vi "FPGA Read.vi"(8 "error in (no error)":errorcluster, 11 "FPGA VI Reference IN":refnum<k20>) -> (0 "error out":errorcluster, 1 "DIO OUT":bool[](array[boolean]), 2 "Raw Ball Voltages OUT":sgl[](array[numeric]), 3 "FPGA VI Reference OUT":refnum<k20>)   [LabVIEW 2018]
uses:
  <vilib>/Utility/error.llb/Error Cluster From Error Code.vi
  <vilib>/rvi/errors/niLvFpgaAdjustHostInterfaceError.vi
  <vilib>/rvi/interface/nirviReadWriteControl/nirviReadWriteControl.xnode
  NiFpgaLv.dll
  <vilib>/rvi/interface/Simulation/niFpgaSimulationCallBeginRW.vi
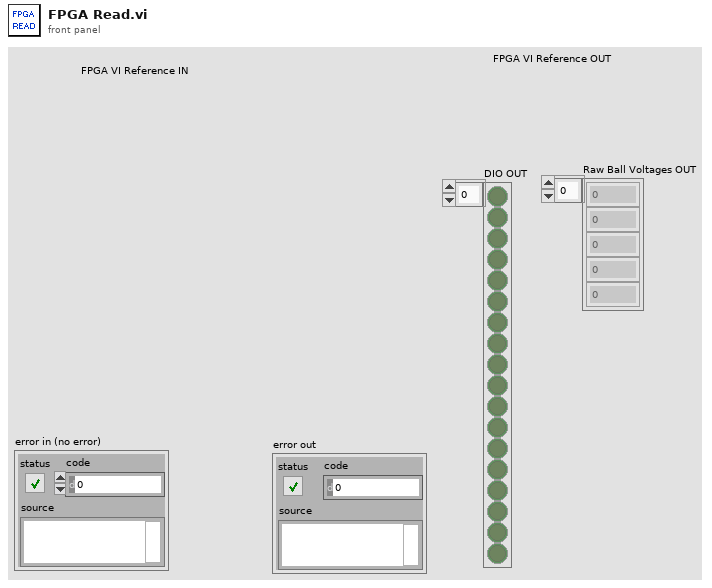
[diagram p1: front panel]
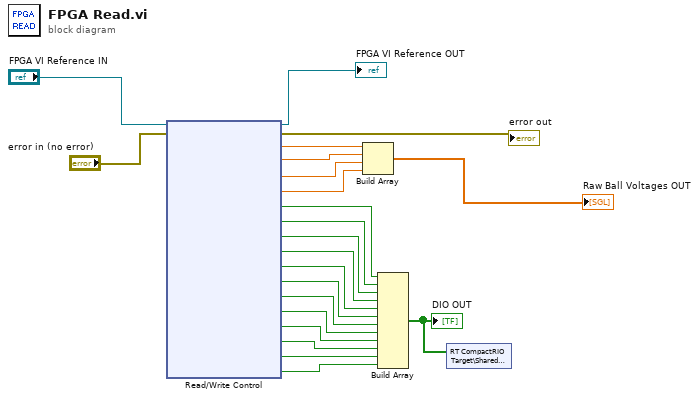
[diagram p0: block diagram]
diagram:
  n1 = xnode "Read/Write Control"("FPGA VI Reference In"="FPGA VI Reference IN", "error in"="error in (no error)") -> ("FPGA VI Reference Out"=→"FPGA VI Reference OUT":refnum<k20>, "error out"=→"error out":errorcluster, "Vx0"=w18:sgl, "Vy0"=w19:sgl, "Vx1"=w20:sgl, "Vy1"=w21:sgl, "aClck_DI"=w4:bool, "frame_clock_DO"=w5:bool, "whisker_video_ctrl"=w6:bool, "lick_signal_DI"=w7:bool, "water_valve_ctrl"=w8:bool, "laser_ctrl"=w9:bool, "left_texture_ctrl"=w10:bool, "right_texture_ctrl"=w11:bool, "trial_ephys_ctrl"=w12:bool, "trial_iti_ctrl_DO"=w13:bool, "trial_on_ctrl_DO"=w14:bool, "ephys_clock_DO"=w17:bool)
  n2 = Build Array(w18, w19, w20, w21) -> (→"Raw Ball Voltages OUT":sgl[])
  n3 = Build Array(w4, w5, w6, w7, w8, w9, w10, w11, w12, w13, w14, w17) -> (w3:bool[])
  "DIO OUT" <- w3
  n4 = shared-variable "RT CompactRIO Target\\Shared Variables.lvlib\\DIO"(w3) -> ()  [unwired: 1 in, 1 out]
